vi "Launch_Actor_Test.vi"(8 "error in (no error)":errorcluster caption="entrée d'erreur (pas d'erreur)", 11 "Name Actor":string) -> (0 "error out":errorcluster caption="sortie d'erreur", 1 "Stopped":bool, 2 "Results":bool[](array[boolean]), 3 "Tableau":T3(array[cluster]))   [LabVIEW 2020, in "Library Core.lvlib" / "Actor Test (Default).lvclass"]
uses:
  Actor Test (Default).lvclass
  Commun VI/TypeDef/Commande Test/Commande Value Type.ctl
  Commun VI/TypeDef/Commande Test/Commande Type Test.ctl
  Commun VI/Library Commun.lvlib
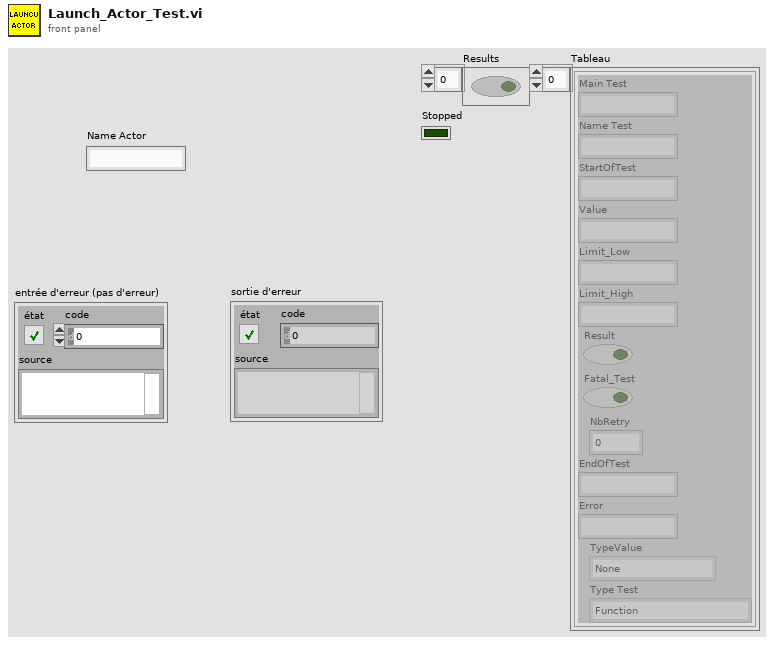
[diagram p1: front panel]
types:
  T1 = typedef "Library Commun.lvlib/Commande Value Type.ctl" = enum16{"None", "String", "Number", "Timestamp", "Boolean", "Array"}
  T2 = typedef "Library Commun.lvlib/Commande Type Test.ctl" = enum16{"Function", "Test", "Calculation"}
  T3 = cluster{"Main Test":string, "Name Test":string, "StartOfTest":string, "Value":string, "Limit_Low":string, "Limit_High":string, "Result":bool, "Fatal_Test":bool, "NbRetry":dbl, "EndOfTest":string, "Error":string, "TypeValue":T1, "Type Test":T2}[]
  T4 = enum16{"Get Actor Class", "Set Actor object", "Get Actor object", "List Actor", "Init"}
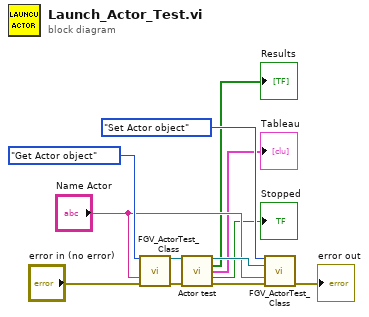
[diagram p0: block diagram]
diagram:
  n1 = call "FGV_ActorTest_Class.vi"("Action"=T4."Get Actor object", "Group Name"="Name Actor", "error in (no error)"="error in (no error)") -> ("Actor Test"=w11:refnum<class "Actor Test (Default).lvclass">, "error out"=w9:errorcluster)  [unwired: 9 in, 2 out]
  n2 = call "Actor test.vi"("Class Actor Test IN"=w11, "entrée d'erreur (pas d'erreur)"=w9) -> ("Class Actor Test Out"=w5:refnum<class "Actor Test (Default).lvclass">, "Results"=→"Results":bool[], "Tableau"=→"Tableau":T3, "Stopped"=→"Stopped":bool, "sortie d'erreur"=w8:errorcluster)  [unwired: 9 in]
  n3 = call "FGV_ActorTest_Class.vi"("Action"=T4."Set Actor object", "Actor Test"=w5, "Group Name"="Name Actor", "error in (no error)"=w8) -> ("error out"=→"error out":errorcluster)  [unwired: 8 in, 3 out]
